vi "Broadcast Mouse Move.vi"(8 "error in (no error)":errorcluster, 10 "Mouse Move":T1, 11 "Map View in":refnum<class "Map View.lvclass">) -> (0 "error out":errorcluster, 3 "Map View out":refnum<class "Map View.lvclass">)   [LabVIEW 2020, in "Map View.lvlib" / "Map View.lvclass"]
uses:
  Map View.lvclass
  <vilib>/Utility/miscctls.llb/LVPoint32TypeDef.ctl
  Map View Messages/Abstract Mouse Move Msg/Abstract Mouse Move Msg.lvclass
  C:/Program Files/National Instruments/LabVIEW 2020/vi.lib/ActorFrameworkObserver/Data Message/Data Message.lvclass
  Map View.lvclass/Map View.ctl
  <vilib>/ActorFrameworkObserver/Actor Register/Actor Register.lvclass
panel:
  # "NOTICE -- YOU MUST LEAVE THIS NOTICE IN PLACE.\n\nCopyright (c) 2017, LIANG LIU Shawn.Liu.cn@gmail.com\nAll rights reserved.\n\nRedistribution and use in source and binary forms, with or without modification, are permitted provided that the following conditions are met:\n-Redistributions of source code must retain the above copyright notice, this list of conditions and the following disclaimer.\n-Redistributions in binary form must reproduce the above copyright notice, this list of conditions and the following disclaimer in the documentation and/or other materials provided with the distribution.\n-Neither the name of the eLp nor the names of its contributors may be used to endorse or promote products derived from this software without specific prior written permission.\n\nTHIS SOFTWARE IS PROVIDED BY THE COPYRIGHT HOLDERS AND CONTRIBUTORS \"AS IS\" AND ANY EXPRESS OR IMPLIED WARRANTIES, INCLUDING, BUT NOT LIMITED TO, THE IMPLIED WARRANTIES OF MERCHANTABILITY AND FITNESS FOR A PARTICULAR PURPOSE ARE DISCLAIMED. IN NO EVENT SHALL THE COPYRIGHT HOLDER OR CONTRIBUTORS BE LIABLE FOR ANY DIRECT, INDIRECT, INCIDENTAL, SPECIAL, EXEMPLARY, OR CONSEQUENTIAL DAMAGES (INCLUDING, BUT NOT LIMITED TO, PROCUREMENT OF SUBSTITUTE GOODS OR SERVICES; LOSS OF USE, DATA, OR PROFITS; OR BUSINESS INTERRUPTION) HOWEVER CAUSED AND ON ANY THEORY OF LIABILITY, WHETHER IN CONTRACT, STRICT LIABILITY, OR TORT (INCLUDING NEGLIGENCE OR OTHERWISE) ARISING IN ANY WAY OUT OF THE USE OF THIS SOFTWARE, EVEN IF ADVISED OF THE POSSIBILITY OF SUCH DAMAGE."
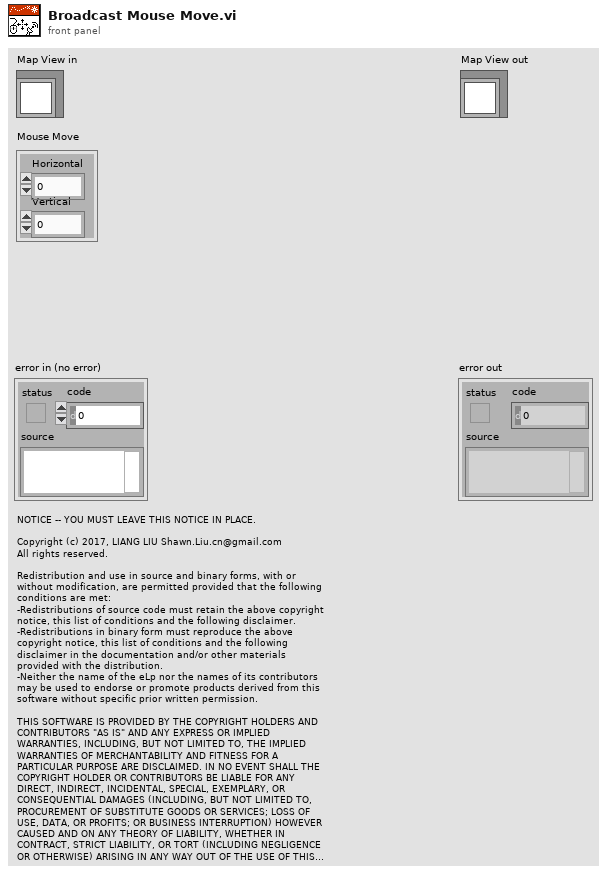
[diagram p1: front panel]
types:
  T1 = typedef "LVPoint32TypeDef.ctl" = cluster{"Horizontal":i32, "Vertical":i32}
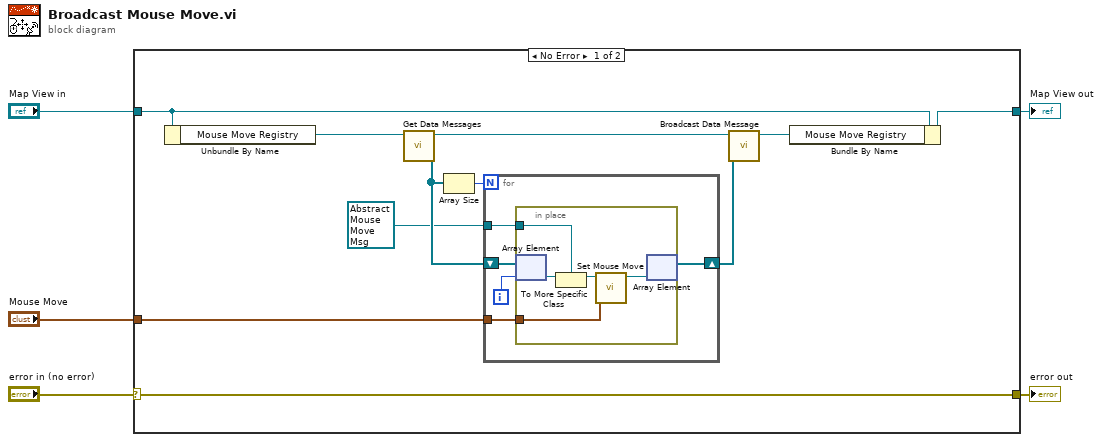
[diagram p0: block diagram]
diagram:
  n1 = case "Error Case" shown="No Error" "error in (no error)" {
    selector: "error in (no error)" -> [w7 w28]
    tunnel: "Map View in" -> [w16 w27]
    tunnel: [w15 w27] -> w4
    tunnel: [w7 w28] -> w3
    tunnel: "Mouse Move" -> [w6 _]
    frame No Error {
      n2 = Unbundle By Name(w16) -> ("Mouse Move Registry"=w14:refnum<class "Actor Register.lvclass">)
      n3 = call-dynamic "Get Data Messages.vi"("Actor Register in"=w14) -> ("Data Messages"=w11:refnum<class "Data Message.lvclass">[], "Actor Register out"=w13:refnum<class "Actor Register.lvclass">)  [unwired: 9 in]
      n4 = Array Size(array=w11) -> (size(s)=w9:i32)
      n5 = for {
        N: w9 -> [_]
        shift-right: [w19] -> w8
        shift-left: w11 -> [w21]
        tunnel: refnum<class "Abstract Mouse Move Msg.lvclass"> refnum ("Map View.lvlib:Abstract Mouse Move Msg.lvclass") -> [w20]
        tunnel: w6 -> [w17]
        i -> [w18]
        n6 = in-place {
          in-place-border: w20 -> [w25]
          in-place-border: w17 -> [w22]
          n7 = in-place-array #1(w21, w18) -> (w26:refnum<class "Data Message.lvclass">)
          n8 = To More Specific Class(target class=w25, reference=w26) -> (specific class reference=w24:refnum<class "Abstract Mouse Move Msg.lvclass">)  [unwired: 1 in, 1 out]
          n9 = call "Set Mouse Move.vi"("Mouse Move"=w22, "Abstract Mouse Move Msg in"=w24) -> ("Abstract Mouse Move Msg out"=w23:refnum<class "Abstract Mouse Move Msg.lvclass">)  [unwired: 9 in]
          n10 = in-place-array #1(w23) -> (w19:refnum<class "Data Message.lvclass">[])  [unwired: 1 out]
        }
      }
      n11 = call <vilib>:"Broadcast Data Message.vi"("Data Messages"=w8, "Actor Register in"=w13) -> ("Actor Register out"=w12:refnum<class "Actor Register.lvclass">)  [unwired: 8 in, 1 out]
      n12 = Bundle By Name(cluster=w16, "Mouse Move Registry"=w12) -> (w15:refnum<class "Map View.lvclass">)
    }
    frame Error {
    }
  }
  "error out" <- w3
  "Map View out" <- w4
